vi "Sans titre 2.vi"() -> ()   [LabVIEW 2026]
panel:
  in  "save variables":bool
  in  "stop":bool
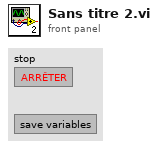
[diagram p1: front panel]
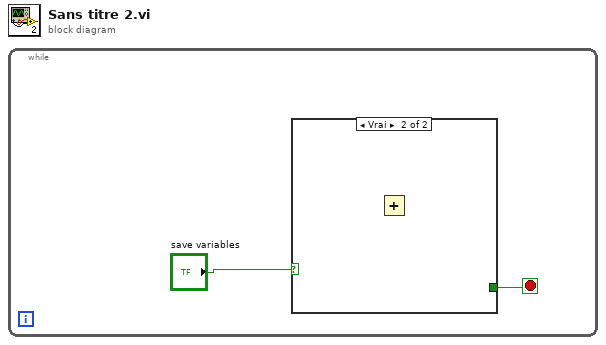
[diagram p0: block diagram]
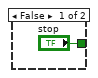
[diagram p2: hidden frame]
diagram:
  n1 = while {
    stop <- w2 stop-if-true
    n2 = case shown="Vrai" "save variables" {
      tunnel: ["stop" _] -> w2
      frame False {
      }
      frame True {
        n3 = Add() -> ()  [unwired: 2 in, 1 out]
      }
    }
  }
